vi "Newport_mono.vi"(3 "Go to Wavelength":dbl format="%.4f") -> (0 "Current Wavelength":dbl format="%.4f")   [LabVIEW 2017]
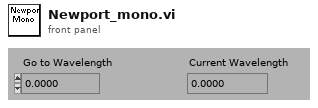
[diagram p1: front panel]
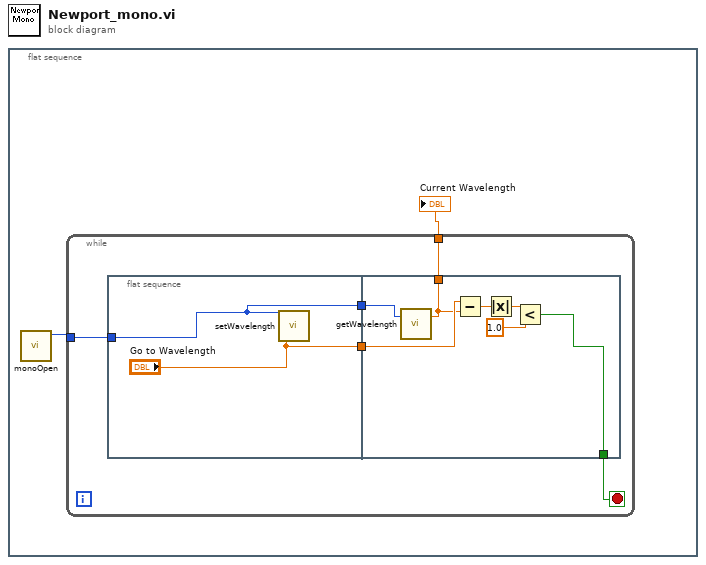
[diagram p0: block diagram]
diagram:
  n1 = flat-sequence {
    frame #0 {
      n2 = call "monoOpen.vi"() -> ("Mono0ID"=w1:u32)  [unwired: 10 in, 1 out]
      n3 = while {
        tunnel: [w4] -> w2
        tunnel: w1 -> [w3]
        stop <- w5 stop-if-true
        n4 = flat-sequence {
          tunnel: [w8] -> w7
          tunnel: ["Go to Wavelength"] -> w6
          tunnel: w3 -> [w8]
          tunnel: w7 -> [w16]
          tunnel: w6 -> [w15]
          tunnel: [w10] -> w5
          tunnel: [w11] -> w4
          frame #0 {
            n5 = call "setWavelength.vi"("Destination Wavelength"="Go to Wavelength", "Mono Numbers"=w8) -> ()  [unwired: 1 in, 1 out]
          }
          frame #1 {
            n6 = call "getWavelength.vi"("Mono Numbers"=w16) -> ("Present Wavelength"=w11:dbl)  [unwired: 1 in, 1 out]
            n7 = Subtract(x=w15, y=w11) -> (x-y=w14:dbl)
            n8 = Absolute Value(x=w14) -> (abs(x)=w13:dbl)
            n9 = Less?(x=w13, y=1.0) -> (x < y?=w10:bool)
          }
        }
      }
      "Current Wavelength" <- w2
    }
  }
